vi "formatPointData.vi"(11 "point":T1[](array[typedef])=[{"X"=0.0, "Y"=0.0, "Z"=0.0}, {"X"=0.0, "Y"=0.0, "Z"=0.0}]) -> (3 "formatedPointData":string)   [LabVIEW 2015]
uses:
  <vilib>/Utility/miscctls.llb/LV3DPointTypeDef.ctl
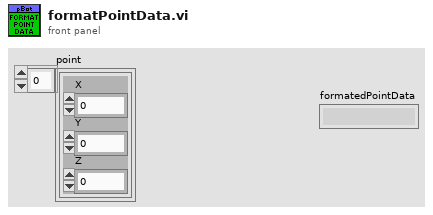
[diagram p1: front panel]
types:
  T1 = typedef "LV3DPointTypeDef.ctl" = cluster{"X":sgl, "Y":sgl, "Z":sgl}
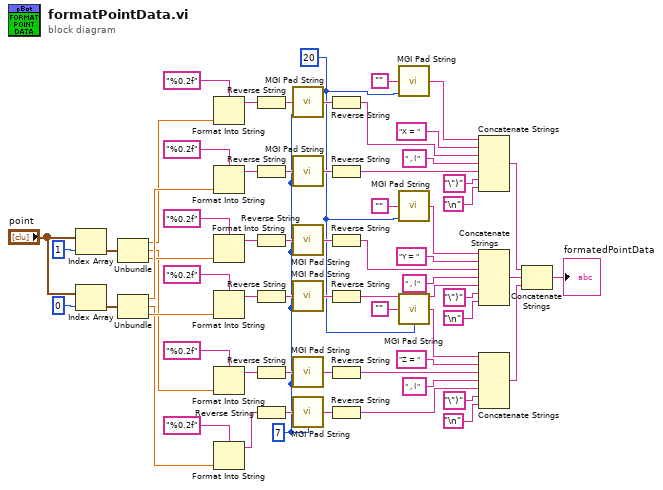
[diagram p0: block diagram]
diagram:
  w4 = u32 7 ("End Length")
  w1 = u32 20 ("End Length")
  n1 = Index Array(array="point", index=1) -> (element=w55:T1)
  n2 = Index Array(array="point", index=0) -> (element=w54:T1)
  n3 = Unbundle(w55) -> ("X"=w42:sgl, "Y"=w6:sgl, "Z"=w8:sgl)
  n4 = Unbundle(w54) -> ("X"=w62:sgl, "Y"=w5:sgl, "Z"=w7:sgl)
  n5 = Format Into String(format string="%0.2f", w42) -> (resulting string=w44:string)  [unwired: 2 in, 1 out]
  n6 = Format Into String(format string="%0.2f", w62) -> (resulting string=w51:string)  [unwired: 2 in, 1 out]
  n7 = Format Into String(format string="%0.2f", w8) -> (resulting string=w38:string)  [unwired: 2 in, 1 out]
  n8 = Format Into String(format string="%0.2f", w7) -> (resulting string=w31:string)  [unwired: 2 in, 1 out]
  n9 = Format Into String(format string="%0.2f", w6) -> (resulting string=w11:string)  [unwired: 2 in, 1 out]
  n10 = Format Into String(format string="%0.2f", w5) -> (resulting string=w18:string)  [unwired: 2 in, 1 out]
  n11 = Reverse String(1:w44) -> (0:w45:string)
  n12 = Reverse String(1:w51) -> (0:w50:string)
  n13 = Reverse String(1:w38) -> (0:w37:string)
  n14 = Reverse String(1:w31) -> (0:w32:string)
  n15 = Reverse String(1:w11) -> (0:w12:string)
  n16 = Reverse String(1:w18) -> (0:w17:string)
  n17 = call <userlib>:"MGI Pad String.vi"("String In"=w45, "End Length"=w4) -> ("String Out"=w46:string)  [unwired: 13 in]
  n18 = call <userlib>:"MGI Pad String.vi"("String In"=w50, "End Length"=w4) -> ("String Out"=w49:string)  [unwired: 13 in]
  n19 = call <userlib>:"MGI Pad String.vi"("String In"=w37, "End Length"=w4) -> ("String Out"=w36:string)  [unwired: 13 in]
  n20 = call <userlib>:"MGI Pad String.vi"("String In"=w32, "End Length"=w4) -> ("String Out"=w33:string)  [unwired: 13 in]
  n21 = call <userlib>:"MGI Pad String.vi"("String In"=w12, "End Length"=w4) -> ("String Out"=w13:string)  [unwired: 13 in]
  n22 = call <userlib>:"MGI Pad String.vi"("String In"=w17, "End Length"=w4) -> ("String Out"=w16:string)  [unwired: 13 in]
  n23 = Reverse String(1:w46) -> (0:w41:string)
  n24 = Reverse String(1:w49) -> (0:w48:string)
  n25 = Reverse String(1:w36) -> (0:w40:string)
  n26 = Reverse String(1:w33) -> (0:w34:string)
  n27 = Reverse String(1:w13) -> (0:w9:string)
  n28 = Reverse String(1:w16) -> (0:w15:string)
  n29 = call <userlib>:"MGI Pad String.vi"("String In"="", "End Length"=w1) -> ("String Out"=w64:string)  [unwired: 13 in]
  n30 = call <userlib>:"MGI Pad String.vi"("String In"="", "End Length"=w1) -> ("String Out"=w26:string)  [unwired: 13 in]
  n31 = call <userlib>:"MGI Pad String.vi"("String In"="", "End Length"=w1) -> ("String Out"=w23:string)  [unwired: 13 in]
  n32 = Concatenate Strings(w64, "X = " ("format string"), w41, " , (" ("string"), w48, "\")" ("string"), "\n") -> (w53:string)
  n33 = Concatenate Strings(w26, "Y = " ("format string"), w40, " , (" ("string"), w34, "\")" ("string"), "\n") -> (w3:string)
  n34 = Concatenate Strings(w23, "Z = " ("format string"), w9, " , (" ("string"), w15, "\")" ("string"), "\n") -> (w2:string)
  n35 = Concatenate Strings(w53, w3, w2) -> (→"formatedPointData":string)
